vi "Expert_SetDevice.vi"(0 "ID Device":i32, 7 "Error IN Toolkit":i32, 11 "Error In LabVIEW":errorcluster) -> (8 "Error OUT Toolkit":i32, 15 "Error OUT LabVIEW":errorcluster)   [LabVIEW 2018]
doc: "It sets as the device GPU to use when passing its identifier. It receives an integer identifier and in case this VI is not initial, it receives an error integer from a VI that uses the same DLL to avoid errors."
uses:
  dll/LibreriaAutis_3.dll
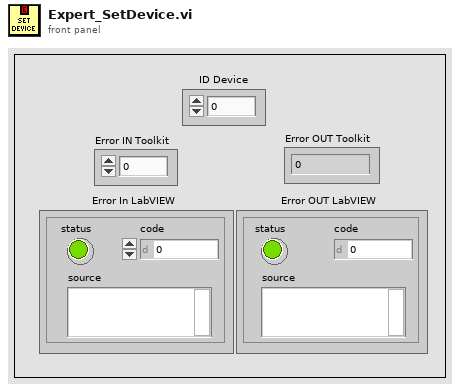
[diagram p1: front panel]
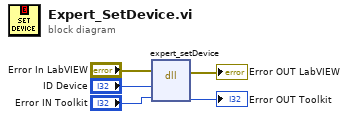
[diagram p0: block diagram]
diagram:
  n1 = dll-call lib="C:/Users/AUTIS/Desktop/LibreriaAUTIS/LabVIEW/dll/LibreriaAutis_3.dll" fn="expert_setDevice"(error in="Error In LabVIEW", "deviceId"="ID Device", "error"="Error IN Toolkit") -> (error out=→"Error OUT LabVIEW":errorcluster, "error"=→"Error OUT Toolkit":i32)  [unwired: 4 in, 1 out]
